vi "Get Joystick Axes.vi"(11 "Axes":T1) -> (1 "Numeric":dbl, 2 "joystick out":dbl, 3 "joystick out 2":dbl)   [LabVIEW 2012]
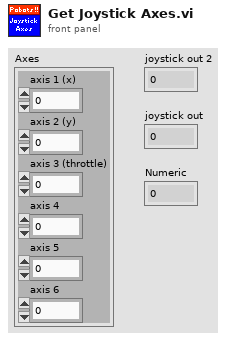
[diagram p1: front panel]
types:
  T1 = cluster{"axis 1 (x)":dbl, "axis 2 (y)":dbl, "axis 3 (throttle)":dbl, "axis 4":dbl, "axis 5":dbl, "axis 6":dbl}
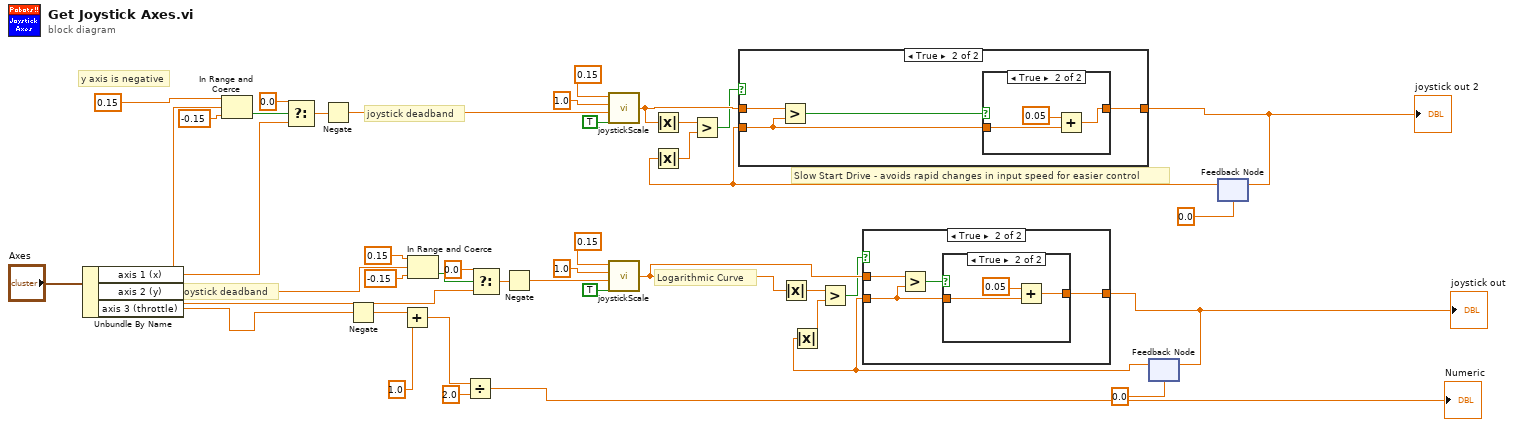
[diagram p0: block diagram]
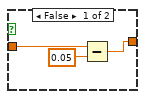
[diagram p3: hidden frame]
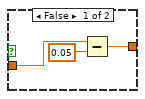
[diagram p5: hidden frame]
diagram:
  # "joystick deadband"
  # "y axis is negative"
  # "joystick deadband"
  # "Logarithmic Curve"
  # "Slow Start Drive - avoids rapid changes in input speed for easier control"
  n1 = Unbundle By Name("Axes") -> ("axis 1 (x)"=w1:dbl, "axis 2 (y)"=w2:dbl, "axis 3 (throttle)"=w41:dbl)
  n2 = In Range and Coerce(upper limit=0.15, x=w1, lower limit=-0.15) -> (In Range?=w23:bool)  [unwired: 1 out]
  n3 = Select(t=0.0, s=w23, f=w1) -> (s? t:f=w30:dbl)
  n4 = Negate(x=w30) -> (-x=w32:dbl)
  n5 = Negate(x=w41) -> (-x=w36:dbl)
  n6 = Add(x=w36, y=1.0) -> (x+y=w38:dbl)
  n7 = In Range and Coerce(upper limit=0.15, x=w2, lower limit=-0.15) -> (In Range?=w27:bool)  [unwired: 1 out]
  n8 = Divide(x=w38, y=2.0) -> (x/y=→"Numeric":dbl)
  n9 = Select(t=0.0, s=w27, f=w2) -> (s? t:f=w29:dbl)
  n10 = Negate(x=w29) -> (-x=w31:dbl)
  n11 = call "joystickScale.vi"("Logarithmic?"=TRUE, "joystick in"=w32, "max"=1.0, "min"=0.15 ("x min")) -> ("joystick out"=w11:dbl)
  n12 = call "joystickScale.vi"("Logarithmic?"=TRUE, "joystick in"=w31, "max"=1.0, "min"=0.15 ("y min")) -> ("joystick out"=w17:dbl)
  n13 = Absolute Value(x=w11) -> (abs(x)=w9:dbl)
  n14 = Absolute Value(x=w17) -> (abs(x)=w15:dbl)
  n15 = feedback #1(0.0) -> (w14:dbl)
  n16 = Absolute Value(x=w14) -> (abs(x)=w16:dbl)
  n17 = Greater?(x=w15, y=w16) -> (0:w13:bool)
  n18 = case shown="True" w13 {
    tunnel: w14 -> [_ w46]
    tunnel: w17 -> [w42 w44]
    tunnel: [w42 w43] -> w34
    frame False {
    }
    frame True {
      n19 = Greater?(x=w44, y=w46) -> (0:w45:bool)
      n20 = case shown="True" w45 {
        tunnel: [w49 w51] -> w43
        tunnel: w46 -> [w47 w50]
        frame False {
          n21 = Subtract(x=w47, y=0.05) -> (x-y=w49:dbl)
        }
        frame True {
          n22 = Add(x=0.05, y=w50) -> (x+y=w51:dbl)
        }
      }
    }
  }
  "joystick out" <- w34
  n23 = feedback-in #1(w34) -> ()
  n24 = feedback #2(0.0) -> (w8:dbl)
  n25 = Absolute Value(x=w8) -> (abs(x)=w10:dbl)
  n26 = Greater?(x=w9, y=w10) -> (0:w7:bool)
  n27 = case shown="True" w7 {
    tunnel: w8 -> [_ w57]
    tunnel: w11 -> [w53 w55]
    tunnel: [w53 w54] -> w33
    frame False {
    }
    frame True {
      n28 = Greater?(x=w55, y=w57) -> (0:w56:bool)
      n29 = case shown="True" w56 {
        tunnel: [w60 w62] -> w54
        tunnel: w57 -> [w58 w61]
        frame False {
          n30 = Subtract(x=w58, y=0.05) -> (x-y=w60:dbl)
        }
        frame True {
          n31 = Add(x=0.05, y=w61) -> (x+y=w62:dbl)
        }
      }
    }
  }
  "joystick out 2" <- w33
  n32 = feedback-in #2(w33) -> ()
